vi "Frequency Ramp.vi"() -> ()   [LabVIEW 2016]
panel:
  in  "Duration (ms)":dbl
  in  "Total Ramping Time (ms)":dbl=45000000.0
  out "Step Seperation (us)":dbl
  in  "Ramp Duration (us)":dbl=45000000.0
  in  "Step Size (Hz)":dbl
  in  "Max Freq (MHz)":dbl=45000000.0
  in  "Min Freq (MHz)":dbl=45000000.0
  in  "start (T) stop (F)":bool=TRUE
  in  "Amplitude (0-1)":dbl=1.0
  in  "Frequency (MHz)":dbl=350.0 format="%#_6p"
  in  "Select Channel":T1(ring)
  out "appended instruction string":string="dds reset\rdcp spi:CFR1=0x404000\rdcp spi:CFR2=0x80080\rdcp 0 spi:STP0=0x3FFF0000028F5C29\rdcp 1 spi:STP0=0x3FFF0000028F5C29\rdcp 0 spi:DRL=0x147C0118147BC1DB\rdcp 0 spi:DRSS=0xFFFFFFFF00000003\rdcp 0 spi:DRR=0x2D3E\rdcp 0 update:u-d\rdcp 0 update:+d\rdcp 1 spi:DRL=0x147AE148147AE148\rdcp 1 spi:DRSS=0xFFFFFFFF00000000\rdcp 1 spi:DRR=0xFFFF\rdcp 1 update:u-d\rdcp 1 update:+d\rdcp wait:1h:\rdcp wait::DROVER\rdcp 0 spi:DRL=0x147C51F1147C0118\rdcp 0 spi:DRSS=0xFFFFFFFF00000004\rdcp 0 spi:DRR=0x2F2F\rdcp 0 update:u-d\rdcp 0 update:+d\rdcp wait:1h:\rdcp wait::DROVER\rdcp 0 spi:DRL=0x147CB92D147C51F1\rdcp 0 spi:DRSS=0xFFFFFFFF00000017\rdcp 0 spi:DRR=0xD478\rdcp 0 update:u-d\rdcp 0 update:+d\rdcp wait:1h:\rdcp wait::DROVER\rdcp 0 spi:DRL=0x147D3CCC147CB92D\rdcp 0 spi:DRSS=0xFFFFFFFF00000009\rdcp 0 spi:DRR=0x4136\rdcp 0 update:u-d\rdcp 0 update:+d\rdcp wait:1h:\rdcp wait::DROVER\rdcp 0 spi:DRL=0x147DE446147D3CCC\rdcp 0 spi:DRSS=0xFFFFFFFF0000000D\rdcp 0 spi:DRR=0x4A07\rdcp 0 update:u-d\rdcp 0 update:+d\rdcp wait:1h:\rdcp wait::DROVER\rdcp 0 spi:DRL=0x147EB8D6147DE446\rdcp 0 spi:DRSS=0xFFFFFFFF0000002B\rdcp 0 spi:DRR=0xC0EC\rdcp 0 update:u-d\rdcp 0 update:+d\rdcp wait:1h:\rdcp wait::DROVER\rdcp 0 spi:DRL=0x147FC5C3147EB8D6\rdcp 0 spi:DRSS=0xFFFFFFFF00000006\rdcp 0 spi:DRR=0x1547\rdcp 0 update:u-d\rdcp 0 update:+d\rdcp wait:1h:\rdcp wait::DROVER\rdcp 0 spi:DRL=0x148118A1147FC5C3\rdcp 0 spi:DRSS=0xFFFFFFFF0000001C\rdcp 0 spi:DRR=0x4ECD\rdcp 0 update:u-d\rdcp 0 update:+d\rdcp wait:1h:\rdcp wait::DROVER\rdcp 0 spi:DRL=0x1482C174148118A1\rdcp 0 spi:DRSS=0xFFFFFFFF00000049\rdcp 0 spi:DRR=0xA3E0\rdcp 0 update:u-d\rdcp 0 update:+d\rdcp wait:1h:\rdcp wait::DROVER\rdcp 0 spi:DRL=0x1484D2A81482C174\rdcp 0 spi:DRSS=0xFFFFFFFF00000003\rdcp 0 spi:DRR=0x568\rdcp 0 update:u-d\rdcp 0 update:+d\rdcp wait:1h:\rdcp wait::DROVER\rdcp 0 spi:DRL=0x148760AD1484D2A8\rdcp 0 spi:DRSS=0xFFFFFFFF0000008C\rdcp 0 spi:DRR=0xCC25\rdcp 0 update:u-d\rdcp 0 update:+d\rdcp wait:1h:\rdcp wait::DROVER\rdcp 0 spi:DRL=0x148A8111148760AD\rdcp 0 spi:DRSS=0xFFFFFFFF00000049\rdcp 0 spi:DRR=0x56FB\rdcp 0 update:u-d\rdcp 0 update:+d\rdcp wait:1h:\rdcp wait::DROVER\rdcp 0 spi:DRL=0x148E48EB148A8111\rdcp 0 spi:DRSS=0xFFFFFFFF00000004\rdcp 0 spi:DRR=0x3F1\rdcp 0 update:u-d\rdcp 0 update:+d\rdcp wait:1h:\rdcp wait::DROVER\rdcp 0 spi:DRL=0x1492CA77148E48EB\rdcp 0 spi:DRSS=0xFFFFFFFF000000A0\rdcp 0 spi:DRR=0x8447\rdcp 0 update:u-d\rdcp 0 update:+d\rdcp wait:1h:\rdcp wait::DROVER\rdcp 0 spi:DRL=0x149811DB1492CA77\rdcp 0 spi:DRSS=0xFFFFFFFF000000D0\rdcp 0 spi:DRR=0x92C9\rdcp 0 update:u-d\rdcp 0 update:+d\rdcp wait:1h:\rdcp wait::DROVER\rdcp 0 spi:DRL=0x149E2175149811DB\rdcp 0 spi:DRSS=0xFFFFFFFF00000100\rdcp 0 spi:DRR=0x9D59\rdcp 0 update:u-d\rdcp 0 update:+d\rdcp wait:1h:\rdcp wait::DROVER\rdcp 0 spi:DRL=0x14A4EE42149E2175\rdcp 0 spi:DRSS=0xFFFFFFFF000000C7\rdcp 0 spi:DRR=0x6D05\rdcp 0 update:u-d\rdcp 0 update:+d\rdcp wait:1h:\rdcp wait::DROVER\rdcp 0 spi:DRL=0x14AC5D7114A4EE42\rdcp 0 spi:DRSS=0xFFFFFFFF00000019\rdcp 0 spi:DRR=0xC87\rdcp 0 update:u-d\rdcp 0 update:+d\rdcp wait:1h:\rdcp wait::DROVER\rdcp 0 spi:DRL=0x14B4443314AC5D71\rdcp 0 spi:DRSS=0xFFFFFFFF00000021\rdcp 0 spi:DRR=0xF8F\rdcp 0 update:u-d\rdcp 0 update:+d\rdcp wait:1h:\rdcp wait::DROVER\rdcp 0 spi:DRL=0x14BC6A7F14B44433\rdcp 0 spi:DRSS=0xFFFFFFFF0000014D\rdcp 0 spi:DRR=0x9838\rdcp 0 update:u-d\rdcp 0 update:+d\rdcp wait:1h:\rdcp wait::DROVER\rdcp 0 spi:DRL=0x14C490CB14BC6A7F\rdcp 0 spi:DRSS=0xFFFFFFFF0000014D\rdcp 0 spi:DRR=0x9838\rdcp 0 update:u-d\rdcp 0 update:+d\rdcp wait:1h:\rdcp wait::DROVER\rdcp 0 spi:DRL=0x14CC778D14C490CB\rdcp 0 spi:DRSS=0xFFFFFFFF00000021\rdcp 0 spi:DRR=0xF8F\rdcp 0 update:u-d\rdcp 0 update:+d\rdcp wait:1h:\rdcp wait::DROVER\rdcp 0 spi:DRL=0x14D3E6BC14CC778D\rdcp 0 spi:DRSS=0xFFFFFFFF00000019\rdcp 0 spi:DRR=0xC87\rdcp 0 update:u-d\rdcp 0 update:+d\rdcp wait:1h:\rdcp wait::DROVER\rdcp 0 spi:DRL=0x14DAB38914D3E6BC\rdcp 0 spi:DRSS=0xFFFFFFFF000000C7\rdcp 0 spi:DRR=0x6D05\rdcp 0 update:u-d\rdcp 0 update:+d\rdcp wait:1h:\rdcp wait::DROVER\rdcp 0 spi:DRL=0x14E0C32314DAB389\rdcp 0 spi:DRSS=0xFFFFFFFF00000100\rdcp 0 spi:DRR=0x9D59\rdcp 0 update:u-d\rdcp 0 update:+d\rdcp wait:1h:\rdcp wait::DROVER\rdcp 0 spi:DRL=0x14E60A8714E0C323\rdcp 0 spi:DRSS=0xFFFFFFFF000000D0\rdcp 0 spi:DRR=0x92C9\rdcp 0 update:u-d\rdcp 0 update:+d\rdcp wait:1h:\rdcp wait::DROVER\rdcp 0 spi:DRL=0x14EA8C1314E60A87\rdcp 0 spi:DRSS=0xFFFFFFFF000000A0\rdcp 0 spi:DRR=0x8447\rdcp 0 update:u-d\rdcp 0 update:+d\rdcp wait:1h:\rdcp wait::DROVER\rdcp 0 spi:DRL=0x14EE53ED14EA8C13\rdcp 0 spi:DRSS=0xFFFFFFFF00000004\rdcp 0 spi:DRR=0x3F1\rdcp 0 update:u-d\rdcp 0 update:+d\rdcp wait:1h:\rdcp wait::DROVER\rdcp 0 spi:DRL=0x14F1745114EE53ED\rdcp 0 spi:DRSS=0xFFFFFFFF00000049\rdcp 0 spi:DRR=0x56FB\rdcp 0 update:u-d\rdcp 0 update:+d\rdcp wait:1h:\rdcp wait::DROVER\rdcp 0 spi:DRL=0x14F4025514F17451\rdcp 0 spi:DRSS=0xFFFFFFFF0000008C\rdcp 0 spi:DRR=0xCC25\rdcp 0 update:u-d\rdcp 0 update:+d\rdcp wait:1h:\rdcp wait::DROVER\rdcp 0 spi:DRL=0x14F6138A14F40255\rdcp 0 spi:DRSS=0xFFFFFFFF00000003\rdcp 0 spi:DRR=0x568\rdcp 0 update:u-d\rdcp 0 update:+d\rdcp wait:1h:\rdcp wait::DROVER\rdcp 0 spi:DRL=0x14F7BC5D14F6138A\rdcp 0 spi:DRSS=0xFFFFFFFF00000049\rdcp 0 spi:DRR=0xA3E0\rdcp 0 update:u-d\rdcp 0 update:+d\rdcp wait:1h:\rdcp wait::DROVER\rdcp 0 spi:DRL=0x14F90F3B14F7BC5D\rdcp 0 spi:DRSS=0xFFFFFFFF0000001C\rdcp 0 spi:DRR=0x4ECD\rdcp 0 update:u-d\rdcp 0 update:+d\rdcp wait:1h:\rdcp wait::DROVER\rdcp 0 spi:DRL=0x14FA1C2814F90F3B\rdcp 0 spi:DRSS=0xFFFFFFFF00000006\rdcp 0 spi:DRR=0x1547\rdcp 0 update:u-d\rdcp 0 update:+d\rdcp wait:1h:\rdcp wait::DROVER\rdcp 0 spi:DRL=0x14FAF0B814FA1C28\rdcp 0 spi:DRSS=0xFFFFFFFF0000002B\rdcp 0 spi:DRR=0xC0EC\rdcp 0 update:u-d\rdcp 0 update:+d\rdcp wait:1h:\rdcp wait::DROVER\rdcp 0 spi:DRL=0x14FB983214FAF0B8\rdcp 0 spi:DRSS=0xFFFFFFFF0000000D\rdcp 0 spi:DRR=0x4A07\rdcp 0 update:u-d\rdcp 0 update:+d\rdcp wait:1h:\rdcp wait::DROVER\rdcp 0 spi:DRL=0x14FC1BD114FB9832\rdcp 0 spi:DRSS=0xFFFFFFFF00000009\rdcp 0 spi:DRR=0x4136\rdcp 0 update:u-d\rdcp 0 update:+d\rdcp wait:1h:\rdcp wait::DROVER\rdcp 0 spi:DRL=0x14FC830D14FC1BD1\rdcp 0 spi:DRSS=0xFFFFFFFF00000017\rdcp 0 spi:DRR=0xD478\rdcp 0 update:u-d\rdcp 0 update:+d\rdcp wait:1h:\rdcp wait::DROVER\rdcp 0 spi:DRL=0x14FCD3E614FC830D\rdcp 0 spi:DRSS=0xFFFFFFFF00000004\rdcp 0 spi:DRR=0x2F2F\rdcp 0 update:u-d\rdcp 0 update:+d\rdcp wait:1h:\rdcp wait::DROVER\rdcp 0 spi:DRL=0x14FD132314FCD3E6\rdcp 0 spi:DRSS=0xFFFFFFFF00000003\rdcp 0 spi:DRR=0x2D3E\rdcp 0 update:u-d\rdcp 0 update:+d\rdcp wait:1h:\rdcp wait::DROVER\rdcp 0 spi:DRL=0x14FD448E14FD1323\rdcp 0 spi:DRSS=0xFFFFFFFF00000002\rdcp 0 spi:DRR=0x2699\rdcp 0 update:u-d\rdcp 0 update:+d\rdcp wait:1h:\rdcp wait::DROVER\rdcp start\r"
  out "error out":errorcluster={"status"=TRUE, "code"=-1073807339, "source"="VISA Read in FlexDDS-NG_USB_Example.vi"}
  out "read buffer":string
  in  "FlexDDS-NG USB VISA resource name (COM)":refnum<visa-resource-name>="COM5"
  # "Ramp Settings"
  # "Single Frequency"
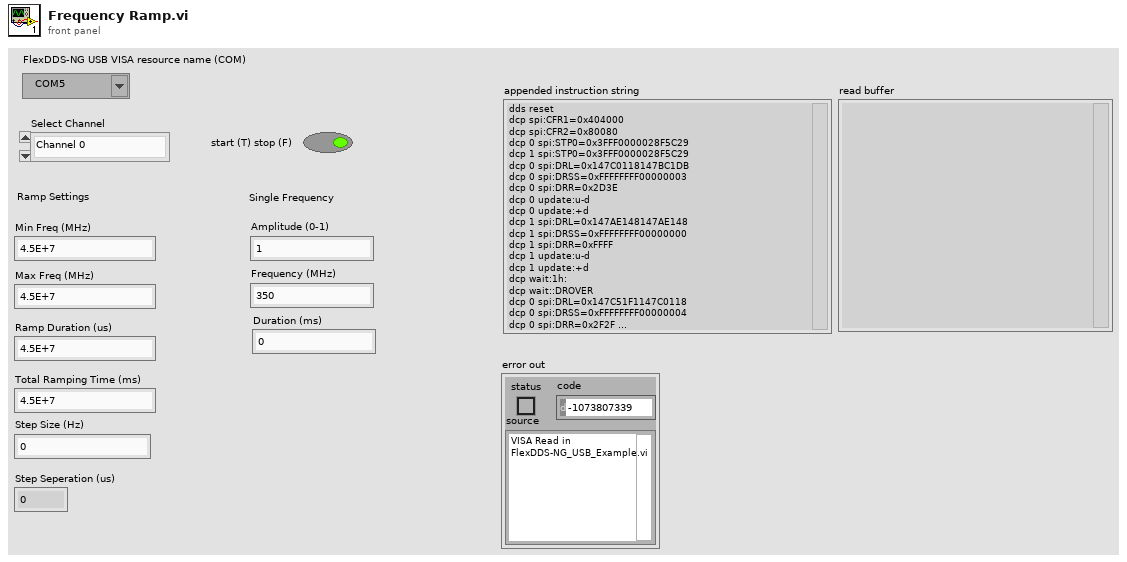
[diagram p1: front panel]
types:
  T1 = enum32{"Channel 0", "Channel 1", "Both channels"}
  T2 = cluster{"Enable ASF from STP (F)":bool, "Digital ramp enable (F)":bool, "Digital ramp no-dwell high (F)":bool, "Digital ramp no-dwell low (F)":bool, "Matched latency enable (T)":bool, "Parallel data port enable (F)":bool}
  T3 = enum16{"no_trigger", "BNC_IN_A_RISING", "BNC_IN_A_FALLING", "BNC_IN_B_RISING", "BNC_IN_B_FALLING", "BNC_IN_C_RISING", "BNC_IN_C_FALLING"}
  T4 = enum32{"O_RAMP_SWP_OVR", "RAM_SWP_OVR", "O_DROVER", "DROVER", "O_SPI_FIFO_EV1", "SPI_FIFO_EV1", "O_SPI_FIFO_EV0", "SPI_FIFO_EV0", "O_SPI_FIFO_FLUSHED", "SPI_FIFO_FLUSHED", "BNC_IN_B_LEVEL", "BNC_IN_B_FALLING", "BNC_IN_B_RISING", "BNC_IN_A_LEVEL", "BNC_IN_A_FALLING", "BNC_IN_A_RISING", "ALL_SPI_FIFOS_FLUSHED", "NONE"}
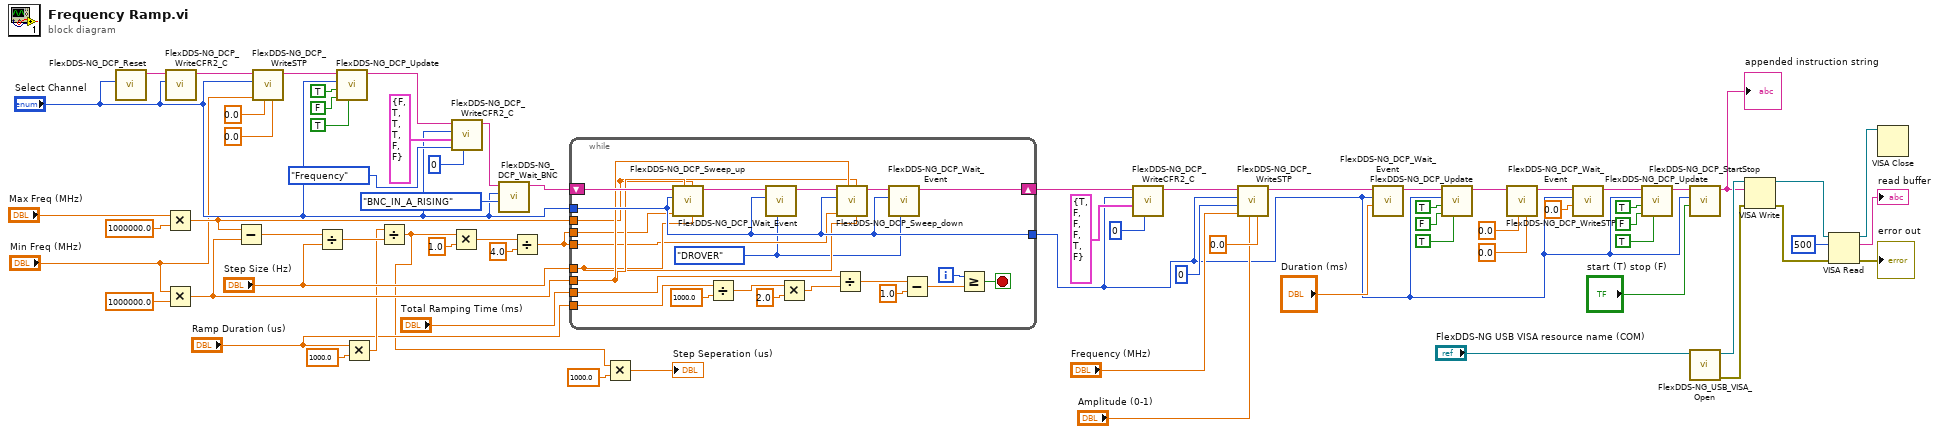
[diagram p0: block diagram]
diagram:
  n1 = call "FlexDDS-NG_DCP_Reset.vi"("Channels"="Select Channel") -> ("appended instruction string"=w26:string)  [unwired: 10 in]
  n2 = Multiply(x="Max Freq (MHz)", y=1000000.0) -> (x*y=w46:dbl)
  n3 = Multiply(x="Min Freq (MHz)", y=1000000.0) -> (x*y=w45:dbl)
  n4 = call "FlexDDS-NG_DCP_WriteCFR2_C.vi"("Channels"="Select Channel", "initial instruction string"=w26) -> ("appended instruction string"=w27:string)  [unwired: 9 in]
  n5 = Subtract(x=w46, y=w45) -> (x-y=w44:dbl)
  n6 = call "FlexDDS-NG_DCP_WriteSTP.vi"("phase degrees (0..360)"=0.0, "amplitude (0..1)"=0.0, "frequency Hz (0..400M)"="Min Freq (MHz)", "Channels"="Select Channel", "initial instruction string"=w27) -> ("appended instruction string"=w28:string)  [unwired: 6 in]
  n7 = Divide(x=w44, y="Step Size (Hz)") -> (x/y=w41:dbl)
  n8 = call "FlexDDS-NG_DCP_Update.vi"("ONLY IO_UPDATE"=TRUE, "DRCTL(true=+, false=-)"=FALSE, "IO_UPDATE(true=u, false = '')"=TRUE, "Channels"="Select Channel", "appended instruction string in"=w28) -> ("appended instruction string out"=w29:string)  [unwired: 6 in]
  n9 = Multiply(x="Ramp Duration (us)", y=1000.0) -> (x*y=w37:dbl)
  n10 = Divide(x=w37, y=w41) -> (x/y=w1:dbl)
  n11 = Multiply(x=w1, y=1.0) -> (x*y=w40:dbl)
  n12 = call "FlexDDS-NG_DCP_WriteCFR2_C.vi"("FM gain (0..15)"=u32 0, "Digital ramp destination"=enum32{"Frequency", "Phase", "Amplitude"}."Frequency", "CFR2 bits"=T2 {"Enable ASF from STP (F)"=FALSE, "Digital ramp enable (F)"=TRUE, "Digital ramp no-dwell high (F)"=TRUE, "Digital ramp no-dwell low (F)"=TRUE, "Matched latency enable (T)"=FALSE, "Parallel data port enable (F)"=FALSE}, "Channels"="Select Channel", "initial instruction string"=w29) -> ("appended instruction string"=w30:string)  [unwired: 6 in]
  n13 = call "FlexDDS-NG_DCP_Wait_BNC.vi"("Trigger"=T3."BNC_IN_A_RISING", "Channels"="Select Channel", "appended instruction string in"=w30) -> ("appended instruction string"=w31:string)  [unwired: 8 in]
  n14 = Divide(x=w40, y=4.0) -> (x/y=w35:dbl)
  n15 = while {
    tunnel: "Select Channel" -> [w91]
    shift-right: [w93] -> w72
    shift-left: w31 -> [w92]
    tunnel: [w91] -> w6
    tunnel: w45 -> [w89]
    tunnel: w46 -> [w88]
    tunnel: "Step Size (Hz)" -> [w87]
    tunnel: w35 -> [w86]
    tunnel: w35 -> [w85]
    tunnel: "Total Ramping Time (ms)" -> [w79]
    tunnel: "Ramp Duration (us)" -> [w84]
    i -> [w76]
    stop <- w74 stop-if-true
    w73 = T4."DROVER" ("Event 1")
    n16 = call "FlexDDS-NG_DCP_Sweep_up.vi"("Step Size (Hz)"=w87, "f1"=w88, "f0"=w89, "Ramp Rate"=w85, "Channels in"=w91, "initial instruction string"=w92) -> ("appended instruction string out"=w90:string)  [unwired: 5 in]
    n17 = Divide(x=w84, y=1000.0) -> (x/y=w82:dbl)
    n18 = call "FlexDDS-NG_DCP_Wait_Event.vi"("Event 1"=w73, "Channels in"=w91, "appended instruction string in"=w90) -> ("appended instruction string"=w95:string)  [unwired: 8 in]
    n19 = Multiply(x=w82, y=2.0) -> (x*y=w80:dbl)
    n20 = Divide(x=w79, y=w80) -> (x/y=w77:dbl)
    n21 = call "FlexDDS-NG_DCP_Sweep_down.vi"("Step Size (Hz)"=w87, "f1"=w88, "f0"=w89, "Ramp Rate"=w86, "Channels in"=w91, "initial instruction string"=w95) -> ("appended instruction string out"=w94:string)  [unwired: 5 in]
    n22 = call "FlexDDS-NG_DCP_Wait_Event.vi"("Event 1"=w73, "Channels in"=w91, "appended instruction string in"=w94) -> ("appended instruction string"=w93:string)  [unwired: 8 in]
    n23 = Subtract(x=w77, y=1.0) -> (x-y=w75:dbl)
    n24 = Greater Or Equal?(x=w76, y=w75) -> (x >= y?=w74:bool)
  }
  n25 = Multiply(x=w1, y=1000.0) -> (x*y=→"Step Seperation (us)":dbl)
  n26 = call "FlexDDS-NG_DCP_WriteCFR2_C.vi"("FM gain (0..15)"=u32 0, "CFR2 bits"=T2 {"Enable ASF from STP (F)"=TRUE, "Digital ramp enable (F)"=FALSE, "Digital ramp no-dwell high (F)"=FALSE, "Digital ramp no-dwell low (F)"=FALSE, "Matched latency enable (T)"=TRUE, "Parallel data port enable (F)"=FALSE}, "Channels"=w6, "initial instruction string"=w72) -> ("appended instruction string"=w71:string)  [unwired: 7 in]
  n27 = call "FlexDDS-NG_DCP_WriteSTP.vi"("phase degrees (0..360)"=0.0, "amplitude (0..1)"="Amplitude (0-1)", "frequency Hz (0..400M)"="Frequency (MHz)", "single tone profile (0..7)"=0, "Channels"=w6, "initial instruction string"=w71) -> ("appended instruction string"=w17:string)  [unwired: 5 in]
  n28 = call "FlexDDS-NG_DCP_Wait_Event.vi"("waiting time [ms]"="Duration (ms)", "Channels in"=w6, "appended instruction string in"=w17) -> ("appended instruction string"=w16:string)  [unwired: 8 in]
  n29 = call "FlexDDS-NG_DCP_Update.vi"("ONLY IO_UPDATE"=TRUE, "DRCTL(true=+, false=-)"=FALSE, "IO_UPDATE(true=u, false = '')"=TRUE, "Channels"=w6, "appended instruction string in"=w16) -> ("appended instruction string out"=w12:string)  [unwired: 6 in]
  n30 = call "FlexDDS-NG_DCP_WriteSTP.vi"("phase degrees (0..360)"=0.0, "amplitude (0..1)"=0.0, "initial instruction string"=w12) -> ("appended instruction string"=w7:string)  [unwired: 8 in]
  n31 = call "FlexDDS-NG_DCP_Wait_Event.vi"("waiting time [ms]"=0.0, "Channels in"=w6, "appended instruction string in"=w7) -> ("appended instruction string"=w8:string)  [unwired: 8 in]
  n32 = call "FlexDDS-NG_DCP_Update.vi"("ONLY IO_UPDATE"=TRUE, "DRCTL(true=+, false=-)"=FALSE, "IO_UPDATE(true=u, false = '')"=TRUE, "Channels"=w6, "appended instruction string in"=w8) -> ("appended instruction string out"=w9:string)  [unwired: 6 in]
  n33 = call "FlexDDS-NG_DCP_StartStop.vi"("start (T) stop (F)"="start (T) stop (F)", "Channels"=w6, "initial instruction string"=w9) -> ("appended instruction string"=w62:string)  [unwired: 8 in]
  "appended instruction string" <- w62
  n34 = call "FlexDDS-NG_USB_VISA_Open.vi"("FlexDDS-NG USB VISA resource name (COM)"="FlexDDS-NG USB VISA resource name (COM)") -> ("error out"=w64:errorcluster, "FlexDDS-NG USB VISA resource name out"=w66:refnum<visa-resource-name>)  [unwired: 9 in]
  n35 = VISA Write(VISA resource name=w66, write buffer=w62, error in (no error)=w64) -> (VISA resource name out=w67:refnum<visa-resource-name>, error out=w63:errorcluster)  [unwired: 1 out]
  n36 = VISA Read(VISA resource name=w67, byte count=u32 500, error in (no error)=w63) -> (VISA resource name out=w70:refnum<visa-resource-name>, read buffer=→"read buffer":string, error out=→"error out":errorcluster)  [unwired: 1 out]
  n37 = VISA Close(VISA resource name=w70) -> ()  [unwired: 1 in, 1 out]
